vi "Camera-SetUp-Acquisition.vi"(9 "Laser Shutter":T1=enum."Off", 10 "Image Size":T4={"H Bin"=1.0, "V Bin"=1.0, "Left"=1.0, "Right"=1024.0, "Top"=1.0, "Bottom"=1024.0} {"V Bin" min=0.0; "H Bin" min=0.0 step=1.0}, 11 "Acquisition Parameters":T5={"Readout Mode"=enum."Image", "Set Acquisition Mode"=enum."Single Scan", "Trigger Mode"=enum."Internal", "Exposure Time (s)"=1.0, "Accumulation Cycle (s)"=1.0, "Kinetic Cycle Time (s)"=1.0, "Number of Kinetics"=1, "Number of Accumulations"=1, "Set VS Speed"=1, "Pixel Rate"=enum."Standard CCD 3 Mhz 14 bits", "V Shift Amplitude"=enum."+1", "Preamp Gain"=enum."1.0"}) -> (0 "Error Out":errorcluster, 1 "File properties":T2, 2 "Image Size Out":T3 {"V Bin" min=0.0; "H Bin" min=0.0 step=1.0}, 3 "Continue with acq?":bool)   [LabVIEW 2014]
uses:
  SubVIs/ctt's/image acquisition 3.ctl
  SubVIs/ctt's/image acquisiton 4.ctl
  SubVIs/ctt's/acquisition control.ctl
  Shutter Control/Shutter SubVis/laser shutters.ctl
  SubVIs/ctt's/image-acquision 2.ctl
  <vilib>/vision/Image Controls.llb/IMAQ Image.ctl
  Shutter Control/Shutter SubVis/control shutters.ctl
  Globals/Initilize Globals.vi
panel:
  in  "High Capacity?":bool
  in  "Shutter":i32(ring) items=["Auto", "Stay Open", "Always Closed"]
  out "Actual Exposure Time (sec)":dbl
  in  "STOP":bool
  in  "Preview":bool
  in  "Go":bool
  in  "Number of preview windows":i32=1
  in  "Set to AOI":bool
  in  "Set to 512 x 300":bool
  in  "Set to Maximum":bool
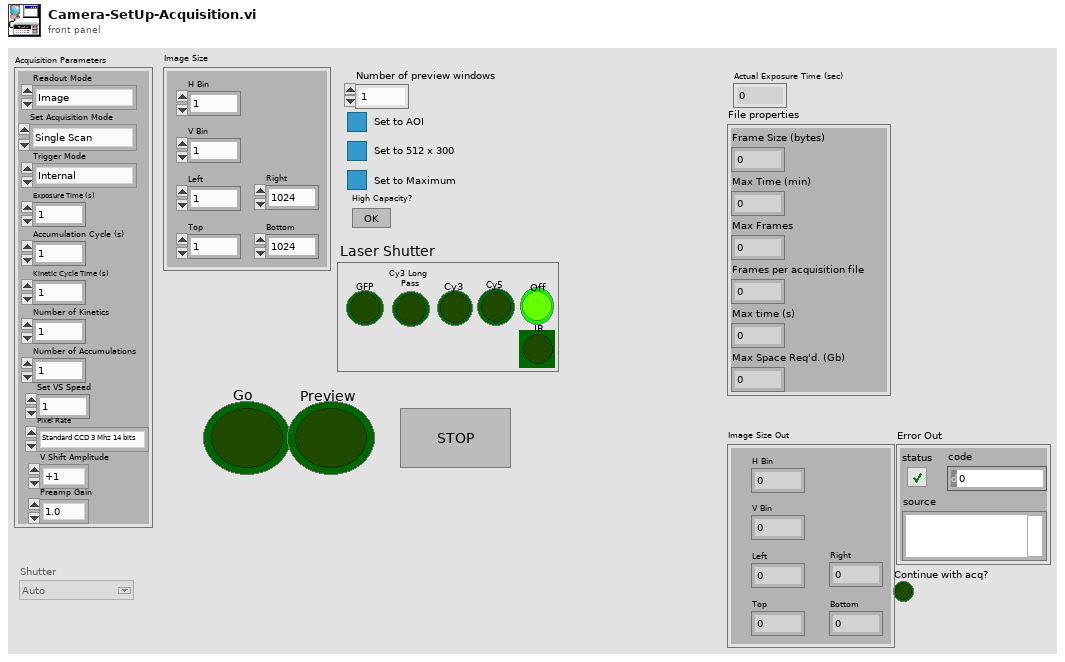
[diagram p1: front panel]
types:
  T1 = typedef "laser shutters.ctl" = enum32{"No Selection", "GFP", "Cy3 Long \nPass", "Cy3", "Cy5", "Off", "IR"}
  T2 = cluster{"Frame Size (bytes)":i32, "Max Time (min)":i32, "Max Frames":i32, "Frames per acquisition file":i32, "Max time (s)":i32, "Max Space Req'd. (Gb)":dbl}
  T3 = typedef "acquisition control.ctl" = cluster{"H Bin":dbl, "V Bin":dbl, "Left":dbl, "Right":dbl, "Top":dbl, "Bottom":dbl}
  T4 = typedef "image acquisiton 4.ctl" = cluster{"H Bin":dbl, "V Bin":dbl, "Left":dbl, "Right":dbl, "Top":dbl, "Bottom":dbl}
  T5 = typedef "image acquisition 3.ctl" = cluster{"Readout Mode":enum16{"Full Vertical Binning", "Multi-Track", "Random-Track", "Single-Track", "Image"}, "Set Acquisition Mode":enum16{"(do nothing)", "Single Scan", "Accumulate", "Kinetics", "Fast Kinetics", "Run till abort"}, "Trigger Mode":enum16{"Internal", "External"}, "Exposure Time (s)":dbl, "Accumulation Cycle (s)":dbl, "Kinetic Cycle Time (s)":dbl, "Number of Kinetics":i32, "Number of Accumulations":i32, "Set VS Speed":i32, "Pixel Rate":enum16{"EM CCD 10 Mhz 14 bits", "EM CCD 5 Mhz 14 bits", "EM CCD 3 Mhz 14 bits", "EM CCD 1 Mhz 16 bits", "Standard CCD 3 Mhz 14 bits", "Standard CCD 1 Mhz 16 bits"}, "V Shift Amplitude":enum16{"normal", "+1", "+2", "+3", "+4"}, "Preamp Gain":enum16{"1.0", "2.4", "5.0"}}
  T6 = typedef "image-acquision 2.ctl" = u32
  T7 = typedef "IMAQ Image.ctl" = refnum<image>
  T8 = typedef "control shutters.ctl" = cluster{"Camera Shutter":bool, "Wheel Speed":u8, "Laser Shutter":enum32{"No Selection", "GFP", "Cy3 Long \nPass", "Cy3", "Cy5", "Off"}}
  T9 = cluster{"H Bin":dbl, "V Bin":dbl, "Left":dbl, "Right":dbl, "Top":dbl, "Bottom":dbl}
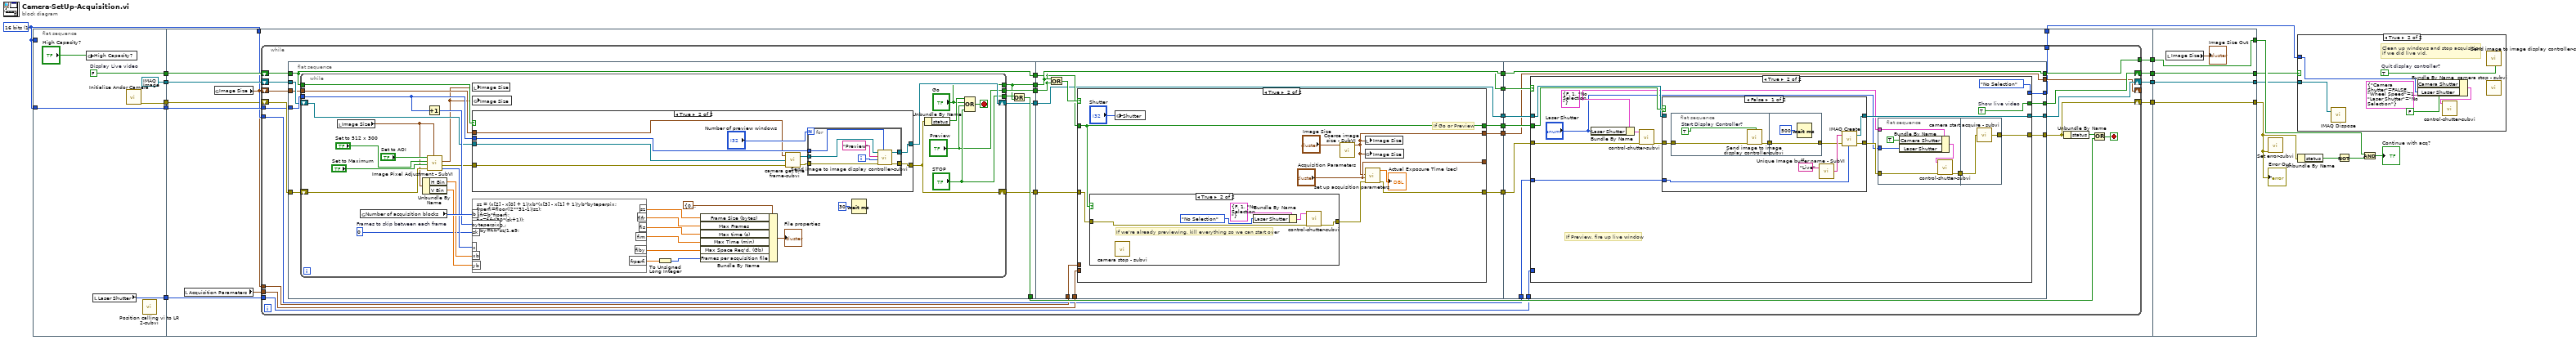
[diagram p0: block diagram]
diagram:
  w2 = T6 1 items=["8 bits", "16 bits", "Float", "Complex", "RGB", "HSL"] ("Image Type")
  n1 = flat-sequence {
    tunnel: [w24] -> w18
    tunnel: [w23] -> w17
    tunnel: w2 -> [w23]
    tunnel: [T7 refnum ("Image")] -> w16
    tunnel: [w19] -> w15
    tunnel: [w20] -> w4
    tunnel: w2 -> [_]
    tunnel: w18 -> [w37]
    tunnel: w17 -> [w36]
    tunnel: w16 -> [w35]
    tunnel: w15 -> [w32]
    tunnel: w2 -> [w33]
    tunnel: [w31] -> w14
    tunnel: [w30] -> w13
    tunnel: [w29] -> w12
    tunnel: [w28] -> w11
    tunnel: w4 -> [w27]
    tunnel: [w25] -> w1
    tunnel: [w217] -> w3
    tunnel: w14 -> [w217]
    tunnel: [w216] -> w6
    tunnel: w13 -> [w216]
    tunnel: [w215] -> w5
    tunnel: w12 -> [w215]
    tunnel: [w214] -> w10
    tunnel: w11 -> [w214]
    frame #0 {
      w24 = FALSE  # Display Live video
      n2 = global write "Initilize Globals.vi" "High Capacity?"("High Capacity?") -> ()
      n3 = local read "Laser Shutter"() -> (w19:T1)
      n4 = call "Initialize Andor Camera.vi"() -> ("Error Out 2"=w20:errorcluster)  [unwired: 10 in, 1 out]
      n5 = call "Position calling vi to LR 2-subvi.vi"() -> ()  [unwired: 4 in, 2 out]
    }
    frame #1 {
      n6 = local read "Acquisition Parameters"() -> (w34:T5)
      n7 = global read "Initilize Globals.vi" "Image Size"() -> (w26:T9)
      n8 = while {
        shift-right: [w44] -> w31
        shift-left: w27 -> [w66]
        shift-right: [w43] -> w30
        shift-left: w37 -> [w65]
        tunnel: w36 -> [w64]
        shift-right: [w42] -> w29
        shift-left: w35 -> [w63]
        shift-right: [w41] -> _
        shift-left: w26 -> [w62]
        tunnel: w26 -> [w52]
        tunnel: w34 -> [w51]
        tunnel: w33 -> [w46]
        tunnel: w32 -> [w45]
        tunnel: [w39] -> w28
        tunnel: [w38] -> w25
        stop <- w59 stop-if-true
        n9 = flat-sequence {
          tunnel: w66 -> [w77]
          tunnel: w65 -> [w68]
          tunnel: w64 -> [w76]
          tunnel: w63 -> [w75]
          tunnel: w62 -> [w74]
          tunnel: [w72] -> w61
          tunnel: [w71] -> w60
          tunnel: [w70] -> w58
          tunnel: [w69] -> w56
          tunnel: [w68] -> w55
          tunnel: [w67] -> w50
          tunnel: w61 -> [w139]
          tunnel: w60 -> [w140]
          tunnel: w56 -> [w134]
          tunnel: w55 -> [w137]
          tunnel: [w140] -> w54
          tunnel: [w139] -> w53
          tunnel: w52 -> [w136]
          tunnel: w51 -> [w135]
          tunnel: w50 -> [w133]
          tunnel: [w133] -> w49
          tunnel: [w132] -> w48
          tunnel: [w131] -> w47
          tunnel: [w130] -> w40
          tunnel: w54 -> [w170]
          tunnel: w53 -> [w171]
          tunnel: w49 -> [w169]
          tunnel: [w170] -> w39
          tunnel: w48 -> [w168]
          tunnel: w47 -> [w167]
          tunnel: w46 -> [w166]
          tunnel: w45 -> [w165]
          tunnel: [w164] -> w44
          tunnel: [w163] -> w43
          tunnel: [w162] -> w42
          tunnel: [w161] -> w38
          tunnel: [w160] -> w41
          tunnel: w40 -> [w160]
          frame #0 {
            n10 = while {
              shift-right: [w88] -> w69
              shift-left: w77 -> [w110]
              tunnel: w68 -> [w93]
              tunnel: w76 -> [w89]
              shift-right: [w87] -> w67
              shift-left: w75 -> [w92]
              tunnel: w74 -> [w91]
              tunnel: ["STOP"] -> w73
              tunnel: ["Go"] -> w71
              tunnel: ["Preview"] -> w72
              stop <- w85 stop-if-true
              w102 = u16 0  # Frames to skip between each frame
              n11 = local read "Image Size"() -> (w79:T4)
              n12 = global read "Initilize Globals.vi" "Number of acquisition blocks"() -> (w106:i8)
              n13 = Unbundle By Name(w79) -> ("H Bin"=w104:dbl, "V Bin"=w103:dbl)
              n14 = Increment(x=w89) -> (x+1=w101:T6)
              n15 = call "Image Pixel Adjustment - SubVI.vi"("Image Size"=w79, "error in"=w110, "Set to Maximum"="Set to Maximum", "Set to 512 x 300"="Set to 512 x 300", "Set to AOI"="Set to AOI") -> ("Pixels Out"=w105:i32[], "Error Out (no error)"=w90:errorcluster, "Image Size 2"=w78:T9)  [unwired: 4 in]
              n16 = local write "Image Size"(w78) -> ()
              n17 = global write "Initilize Globals.vi" "Image Size"(w78) -> ()
              n18 = case shown="True" w93 {
                tunnel: w92 -> [w113 w122]
                tunnel: [w113 w116] -> w87
                tunnel: w91 -> [_ w114]
                tunnel: w90 -> [w112 w121]
                tunnel: w89 -> [_ w117]
                tunnel: [w112 w115] -> w88
                frame False {
                }
                frame True {
                  n19 = call "camera get one frame-subvi.vi"("error in"=w121, "New Image"=w122, "Image Size"=w114) -> ("error out"=w118:errorcluster, "Image Out"=w119:T7)
                  n20 = for {
                    N: "Number of preview windows" -> [_]
                    tunnel: w119 -> [w127]
                    tunnel: w118 -> [w128]
                    tunnel: w117 -> [w129]
                    tunnel: [w124] -> w116
                    tunnel: [w123] -> w115
                    i -> [w125]
                    n21 = call "Send image to image display controller-subvi.vi"("Image"=w127, "Window Title"="Preview" ("Window Title\n(Window only)"), "Window Number"=w125, "error in"=w128, "Image Type"=w129) -> ("Image Out"=w124:T7, "error out"=w123:errorcluster)  [unwired: 4 in]
                  }
                }
              }
              n22 = formula code="sz = (x[2] - x[0] + 1)/xb*(x[3] - x[1] + 1)/yb*byteperpix;\nfrperfi=floor((2**31-1)/sz);\nfifr=b*frperfi;\nfis=fifr/(30*(sk+1));\nfim=fis/60.;\nfiby=fifr*sz/1.e9;"("x"=w105, "b"=w106, "sk"=w102, "xb"=w104, "yb"=w103, "byteperpix"=w101) -> ("sz"=w94:dbl, "fifr"=w95:dbl, "fis"=w96:dbl, "fim"=w97:dbl, "fiby"=w98:dbl, "frperfi"=w100:dbl)
              n23 = To Unsigned Long Integer(number=w100) -> (unsigned 32bit integer=w99:u32)
              n24 = Bundle By Name(cluster=T2 {"Frame Size (bytes)"=0, "Max Time (min)"=0, "Max Frames"=0, "Frames per acquisition file"=0, "Max time (s)"=0, "Max Space Req'd. (Gb)"=0.0}, "Frame Size (bytes)"=w94, "Max Frames"=w95, "Max time (s)"=w96, "Max Time (min)"=w97, "Max Space Req'd. (Gb)"=w98, "Frames per acquisition file"=w99) -> (→"File properties":T2)
              n25 = Wait (ms)(milliseconds to wait=u32 30) -> ()  [unwired: 1 out]
              n26 = Unbundle By Name(w88) -> ("status"=w86:bool)
              n27 = Compound Arithmetic op=OR(w86, "Go", "Preview", "STOP") -> (w85:bool)
            }
            n28 = Or(x=w71, y=w73) -> (x .or. y?=w70:bool)
          }
          frame #1 {
            n29 = Or(x=w140, y=w139) -> (x .or. y?=w138:bool)
            n30 = case shown="True" w138 {
              tunnel: w137 -> [w144 w153]
              tunnel: [w144 w153] -> w131
              tunnel: [w142 "Acquisition Parameters"] -> _
              tunnel: [w143 w145] -> w130
              tunnel: w136 -> [w143 _]
              tunnel: w135 -> [w142 _]
              tunnel: w134 -> [w141 w149]
              tunnel: [w141 w146] -> w132
              frame False {
              }
              frame True {
                # "If Go or Preview"
                n31 = case shown="True" w153 {
                  tunnel: w149 -> [w154 w157]
                  tunnel: [w154 w156] -> w148
                  frame False {
                  }
                  frame True {
                    # "If we're already previewing, kill everything so we can start over"
                    n32 = call "camera stop - subvi.vi"() -> ()  [unwired: 1 in]
                    n33 = Bundle By Name(cluster=T8 {"Camera Shutter"=FALSE, "Wheel Speed"=1, "Laser Shutter"=enum."No Selection"} ("Shutter Control"), "Laser Shutter"=laser_shutters."No Selection" ("Laser Shutter 2")) -> (w155:T8)
                    n34 = call "control-shutter-subvi.vi"("Error In"=w157, "Shutter Control"=w155) -> ("Error Out"=w156:errorcluster)  [unwired: 9 in]
                  }
                }
                n35 = global write "Initilize Globals.vi" "Shutter"("Shutter") -> ()
                n36 = call "Coerce image size - SubVI.vi"("Image Size"="Image Size") -> ("Image Size 2"=w145:T9)  [unwired: 10 in]
                n37 = local write "Image Size"(w145) -> ()
                n38 = global write "Initilize Globals.vi" "Image Size"(w145) -> ()
                n39 = call "set up acquisition parameters.vi"("error in (no error)"=w148, "Acquisition Parameters"="Acquisition Parameters", "Image Size"=w145) -> ("error out"=w146:errorcluster, "Exposure"=→"Actual Exposure Time (sec)":dbl)  [unwired: 2 in, 3 out]
              }
            }
          }
          frame #2 {
            n40 = case shown="True" w171 {
              tunnel: w169 -> [w172 w188]
              tunnel: w168 -> [w175 w180]
              tunnel: w167 -> [w173 w189]
              tunnel: [w175 w183] -> w164
              tunnel: w166 -> [_ w187]
              tunnel: [w173 w186] -> w163
              tunnel: [w174 laser_shutters."No Selection" ("Laser Shutter")] -> w161
              tunnel: w165 -> [w174 _]
              tunnel: [w172 w182] -> w162
              frame False {
              }
              frame True {
                w178 = T8 {"Camera Shutter"=FALSE, "Wheel Speed"=1, "Laser Shutter"=enum."No Selection"} ("Shutter Control")
                w186 = TRUE  # Show live video
                # "If Preview, fire up live window"
                n41 = Bundle By Name(cluster=w178, "Laser Shutter"="Laser Shutter") -> (w181:T8)
                n42 = call "control-shutter-subvi.vi"("Error In"=w180, "Shutter Control"=w181) -> ("Error Out"=w179:errorcluster)  [unwired: 9 in]
                n43 = case shown="False" w189 {
                  tunnel: w179 -> [w205 w211]
                  tunnel: w188 -> [_ w212]
                  tunnel: [w202 w212] -> w182
                  tunnel: [w203 w211] -> w185
                  tunnel: w187 -> [w199 _]
                  frame False {
                    n44 = flat-sequence {
                      tunnel: w205 -> [w208]
                      tunnel: [w206] -> w204
                      tunnel: [w210] -> w198
                      tunnel: w204 -> [w210]
                      frame #0 {
                        w207 = TRUE  # Start Display Controller?
                        n45 = call "Send image to image display controller-subvi.vi"("error in"=w208, "Start display controller?"=w207) -> ("error out"=w206:errorcluster)  [unwired: 7 in, 1 out]
                      }
                      frame #1 {
                        n46 = Wait (ms)(milliseconds to wait=u32 500) -> ()  [unwired: 1 out]
                      }
                    }
                    n47 = call "Unique Image buffer name - SubVI.vi"("Buffer  base name"="Live") -> ("Image Name"=w201:string)  [unwired: 1 in]
                    n48 = call "IMAQ Create"("Image Name"=w201, "Image Type"=w199, "error in (no error)"=w198) -> ("New Image"=w202:T7, "error out"=w203:errorcluster)  [unwired: 1 in, 1 out]
                  }
                  frame True {
                  }
                }
                n49 = flat-sequence {
                  tunnel: w185 -> [w194]
                  tunnel: [w195] -> w184
                  tunnel: w178 -> [w193]
                  tunnel: "Laser Shutter" -> [w192]
                  tunnel: w184 -> [w197]
                  tunnel: [w196] -> w183
                  frame #0 {
                    n50 = Bundle By Name(cluster=w193, "Camera Shutter"=TRUE, "Laser Shutter"=w192) -> (w190:T8)
                    n51 = call "control-shutter-subvi.vi"("Error In"=w194, "Shutter Control"=w190) -> ("Error Out"=w195:errorcluster)  [unwired: 9 in]
                  }
                  frame #1 {
                    n52 = call "camera start acquire - subvi.vi"("error in"=w197) -> ("error out"=w196:errorcluster)
                  }
                }
              }
            }
          }
        }
        n53 = Unbundle By Name(w44) -> ("status"=w57:bool)
        n54 = Or(x=w57, y=w58) -> (x .or. y?=w59:bool)
      }
    }
    frame #2 {
      n55 = local read "Image Size"() -> (→"Image Size Out":T4)
    }
  }
  n56 = call "Set error-subvi.vi"("error in"=w3) -> ()  [unwired: 7 in, 1 out]
  n57 = case shown="True" w6 {
    tunnel: w5 -> [_ w222]
    tunnel: w1 -> [_ w219]
    frame False {
    }
    frame True {
      w223 = TRUE  # Quit display controller?
      # "Clean up windows and stop acquisition\nif we did live vid."
      n58 = call "IMAQ Dispose"("Image"=w222) -> ()  [unwired: 2 in, 4 out]
      n59 = Bundle By Name(cluster=T8 {"Camera Shutter"=FALSE, "Wheel Speed"=1, "Laser Shutter"=enum."No Selection"} ("Shutter Control"), "Camera Shutter"=FALSE, "Laser Shutter"=w219) -> (w220:T8)
      n60 = call "control-shutter-subvi.vi"("Shutter Control"=w220) -> ()  [unwired: 10 in, 1 out]
      n61 = call "Send image to image display controller-subvi.vi"("Quit display controller?"=w223) -> ()  [unwired: 8 in, 2 out]
      n62 = call "camera stop - subvi.vi"() -> ()  [unwired: 1 in]
    }
  }
  n63 = Unbundle By Name(w3) -> ("status"=w9:bool)
  n64 = Not(x=w9) -> (.not. x?=w8:bool)
  n65 = And(x=w10, y=w8) -> (x .and. y?=→"Continue with acq?":bool)
  "Error Out" <- w3
